vi "Read Measurement Data (Occupied Bandwidth).vi"(0 "VISA resource name":refnum<visa-resource-name>, 11 "error in (no error)":errorcluster) -> (4 "VISA resource name out":refnum<visa-resource-name>, 6 "OBW Measurement":T1, 15 "error out":errorcluster)   [LabVIEW 2020, in "Anritsu Signal Analyzer Series.lvlib"]
doc: "Reads Occupied Bandwidth measurement data"
uses:
  Anritsu Signal Analyzer Series.lvlib
panel:
  # "Hz"
  # "Hz"
  # "Hz"
  # "Hz"
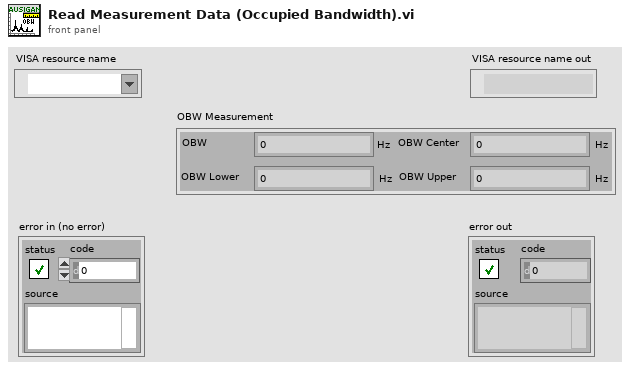
[diagram p1: front panel]
types:
  T1 = cluster{"OBW":dbl, "OBW Center":dbl, "OBW Lower":dbl, "OBW Upper":dbl}
  T2 = cluster{"Values[0]":dbl, "Values[1]":dbl, "Values[2]":dbl, "Values[3]":dbl}
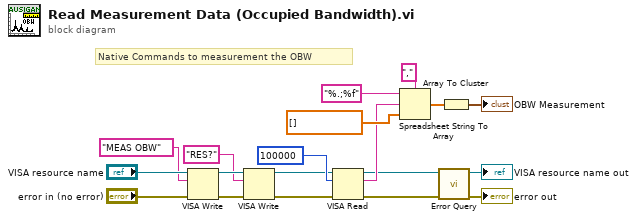
[diagram p0: block diagram]
diagram:
  # "Native Commands to measurement the OBW"
  n1 = VISA Write(VISA resource name="VISA resource name", write buffer="MEAS OBW" ("_CommandSet"), error in (no error)="error in (no error)") -> (VISA resource name out=w8:refnum<visa-resource-name>, error out=w7:errorcluster)  [unwired: 1 out]
  n2 = VISA Write(VISA resource name=w8, write buffer="RES?" ("_Command"), error in (no error)=w7) -> (VISA resource name out=w9:refnum<visa-resource-name>, error out=w10:errorcluster)  [unwired: 1 out]
  n3 = VISA Read(VISA resource name=w9, byte count=u32 100000 ("byte count (0)"), error in (no error)=w10) -> (VISA resource name out=w5:refnum<visa-resource-name>, read buffer=w6:string, error out=w4:errorcluster)  [unwired: 1 out]
  n4 = Spreadsheet String To Array(delimiter (Tab)=",", format string="%.;%f", spreadsheet string=w6, array type (2D Dbl)=dbl[] [] ("Values")) -> (array=w1:dbl[])
  n5 = call "Error Query.vi"("error in (no error)"=w4, "VISA resource name"=w5) -> ("error out"=→"error out":errorcluster, "VISA resource name out"=→"VISA resource name out":refnum<visa-resource-name>)  [unwired: 6 in, 2 out]
  n6 = Array To Cluster(array=w1) -> (cluster=→"OBW Measurement":T2)
